vi "Turret_Set.vi"   [LabVIEW 2019]
uses:
  Globals/Turret_Globals.vi
  Turret_States.ctl
types:
  T1 = typedef "Turret_States.ctl" = enum16{"Manual_Percent_Voltage", "Manual_Speed_Control", "Auto-Target"}
  T2 = typedef "Turret_Cluster.ctl" = cluster{"Auto-Target?":bool, "Control_State":T1, "Turret_Spin_Speed":dbl, "Turret_Spin_Speed_Control?":bool}
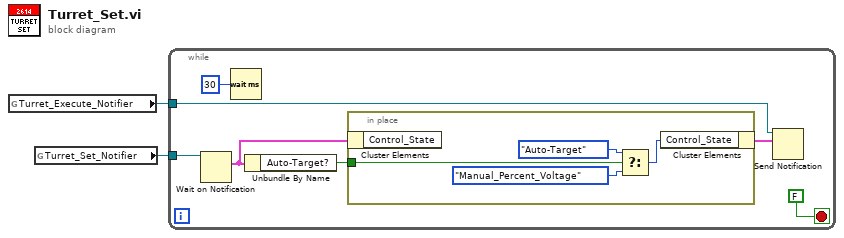
[diagram p0: block diagram]
diagram:
  n1 = global read "Turret_Globals.vi" "Turret_Execute_Notifier"() -> (w1:refnum<notifier>)
  n2 = global read "Turret_Globals.vi" "Turret_Set_Notifier"() -> (w2:refnum<notifier>)
  n3 = while {
    tunnel: w2 -> [w7]
    tunnel: w1 -> [w5]
    stop <- FALSE stop-if-true
    n4 = Wait on Notification(notifier=w7) -> (notification=w4:T2)  [unwired: 3 in, 3 out]
    n5 = Wait (ms)(milliseconds to wait=u32 30) -> ()  [unwired: 1 out]
    n6 = Unbundle By Name(w4) -> ("Auto-Target?"=w3:bool)
    n7 = in-place {
      in-place-border: w3 -> [w13]
      n8 = in-place-cluster #1(w4) -> ()  [unwired: 1 out]
      n9 = Select(t=Turret_States."Auto-Target" ("Control_State"), s=w13, f=Turret_States."Manual_Percent_Voltage" ("Control_State")) -> (s? t:f=w12:T1)
      n10 = in-place-cluster #1("Control_State"=w12) -> (w6:T2)
    }
    n11 = Send Notification(notification=w6, notifier=w5) -> ()  [unwired: 1 in, 2 out]
  }
